vi "InverseOf3x3.vi"() -> ()   [LabVIEW 2015]
panel:
  in  "stop":bool
  out "Inverse of matrix":dbl[][](array[numeric])
  in  "3x3 matrix":dbl[][](array[numeric])
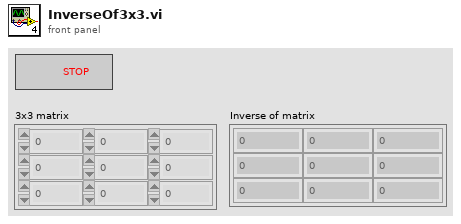
[diagram p1: front panel]
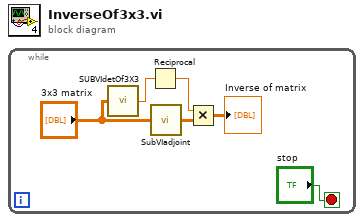
[diagram p0: block diagram]
diagram:
  n1 = while {
    stop <- "stop" stop-if-true
    n2 = call "SUBVIdetOf3X3.vi"("3x3 matrix"="3x3 matrix") -> ("Determinant"=w6:dbl)
    n3 = Reciprocal(x=w6) -> (1/x=w5:dbl)
    n4 = call "SubVIadjoint.vi"("3x3 matrix"="3x3 matrix") -> ("Adjoint of matrix"=w3:dbl[][])
    n5 = Multiply(x=w5, y=w3) -> (x*y=→"Inverse of matrix":dbl[][])
  }
